vi "QWTB Algorithms Filter Find Alg Config.vi"(10 "algorithm name":string, 11 "QWTB path":path) -> (3 "section part":string)   [LabVIEW 2020]
uses:
  octave/infolib/infolib.lvlib
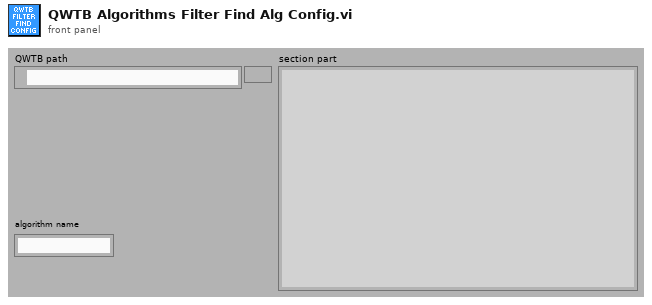
[diagram p1: front panel]
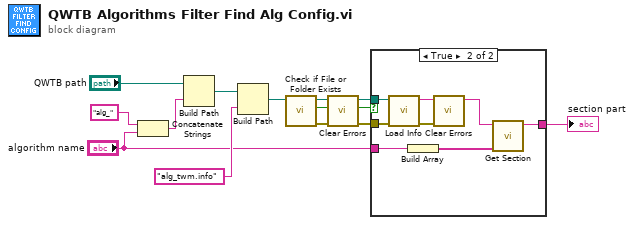
[diagram p0: block diagram]
diagram:
  n1 = Concatenate Strings("alg_" ("string"), "algorithm name") -> (w10:string)
  n2 = Build Path(base path="QWTB path", name or relative path=w10) -> (appended path=w8:path)
  n3 = Build Path(base path=w8, name or relative path="alg_twm.info" ("string")) -> (appended path=w6:path)
  n4 = call <vilib>:"Check if File or Folder Exists.vi"("path"=w6) -> ("error out"=w5:errorcluster, "file or folder exists?"=w9:bool, "dup path"=w4:path)  [unwired: 8 in]
  n5 = call <vilib>:"Clear Errors.vi"("error in (no error)"=w5) -> ("error out"=w3:errorcluster)  [unwired: 5 in, 1 out]
  n6 = case shown="True" w9 {
    tunnel: w4 -> [_ w19]
    tunnel: w3 -> [_ w18]
    tunnel: "algorithm name" -> [_ w16]
    tunnel: [_ w14] -> w1
    frame False {
    }
    frame True {
      n7 = call "Load Info.vi"("error in"=w18, "filename"=w19) -> ("error out"=w13:errorcluster, "info data"=w17:string)  [unwired: 8 in]
      n8 = Build Array(w16) -> (w15:string[])
      n9 = call <vilib>:"Clear Errors.vi"("error in (no error)"=w13) -> ()  [unwired: 5 in, 2 out]
      n10 = call "Get Section.vi"("sections"=w15, "info data"=w17) -> ("section part"=w14:string)  [unwired: 7 in, 2 out]
    }
  }
  "section part" <- w1
